vi "create initialized module for testing.vi"() -> (0 "error out":errorcluster, 1 "2d channels":refnum<class "Profibus channel.lvclass">[][](array[class]), 2 "1d channels":refnum<class "Profibus channel.lvclass">[](array[class]), 3 "Profibus Module configuration out":refnum<class "Profibus Module configuration.lvclass">, 4 "byte orders":T1[](array[typedef])=[{"slave"=1, "big endian"=TRUE}, {"slave"=2, "big endian"=FALSE}, {"slave"=5, "big endian"=TRUE}], 5 "2d names":string[][](array[string]), 6 "slave diagnostics":T2[](array[typedef]), 7 "1d names":string[](array[string]), 8 "RIO interface":string="asd")   [LabVIEW 2013, in "Profibus Module tests.lvlib"]
uses:
  Profibus Module tests.lvlib
  channel/Profibus channel.lvclass
  configuration/Profibus Module configuration.lvclass
  configuration/slave diagnostic configuration.ctl
  <vilib>/NI/Tag Bus Module Framework/channel/TBM channel.lvclass
  configuration/error throw specification.ctl
  configuration/endianness setting.ctl
  <vilib>/NI/Tag Bus/tag/Data Type.ctl
  <vilib>/NI/Tag Bus Module Framework/channel/channel classification.ctl
  configuration/Profibus Module configuration.lvclass/Profibus Module configuration.ctl
  configuration/Write RIO interface.vi
  configuration/Write slave diagnostics.vi
  configuration/Write byte orders.vi
  <vilib>/NI/Tag Bus/tag/tag descriptor.lvclass
  <vilib>/NI/Configuration Framework/serializable configuration/NISE_CEF_serializable configuration.lvclass
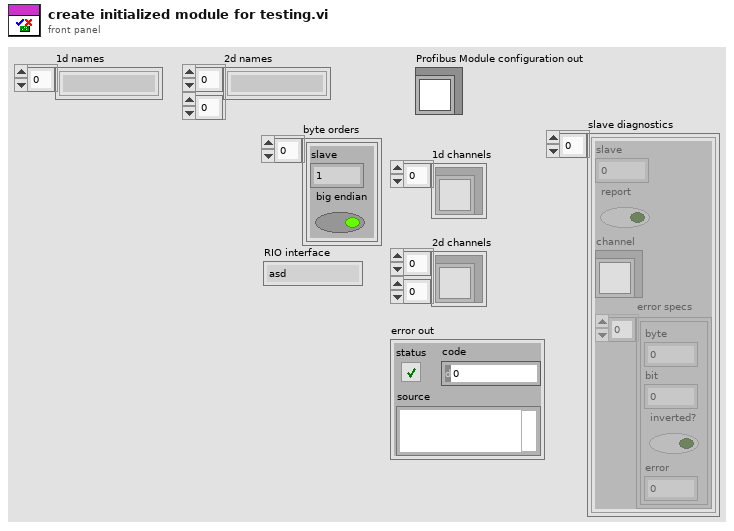
[diagram p1: front panel]
types:
  T1 = typedef "Profibus Module configuration.lvclass/endianness setting.ctl" = cluster{"slave":i8, "big endian":bool}
  T2 = typedef "Profibus Module configuration.lvclass/slave diagnostic configuration.ctl" = cluster{"slave":i8, "report":bool, "channel":refnum<class "TBM channel.lvclass">, "error specs":T3[]}
  T3 = typedef "Profibus Module configuration.lvclass/error throw specification.ctl" = cluster{"byte":i32, "bit":i32, "inverted?":bool, "error":i32}
  T4 = typedef "TBM channel.lvclass/channel classification.ctl" = enum16{"input data", "output data", "processing parameter", "processing result"}
  T5 = typedef "tag bus.lvlib/tag descriptor.lvclass/Data Type.ctl" = enum16{"Double", "Single", "I64", "I32", "I16", "I8", "U64", "U32", "U16", "U8", "Boolean", "String", "Array of Double", "Array of Single", "Array of I64", "Array of I32", "Array of I16", "Array of I8", "Array of U64", "Array of U32", "Array of U16", "Array of U8", "Array of Boolean", "Array of String"}
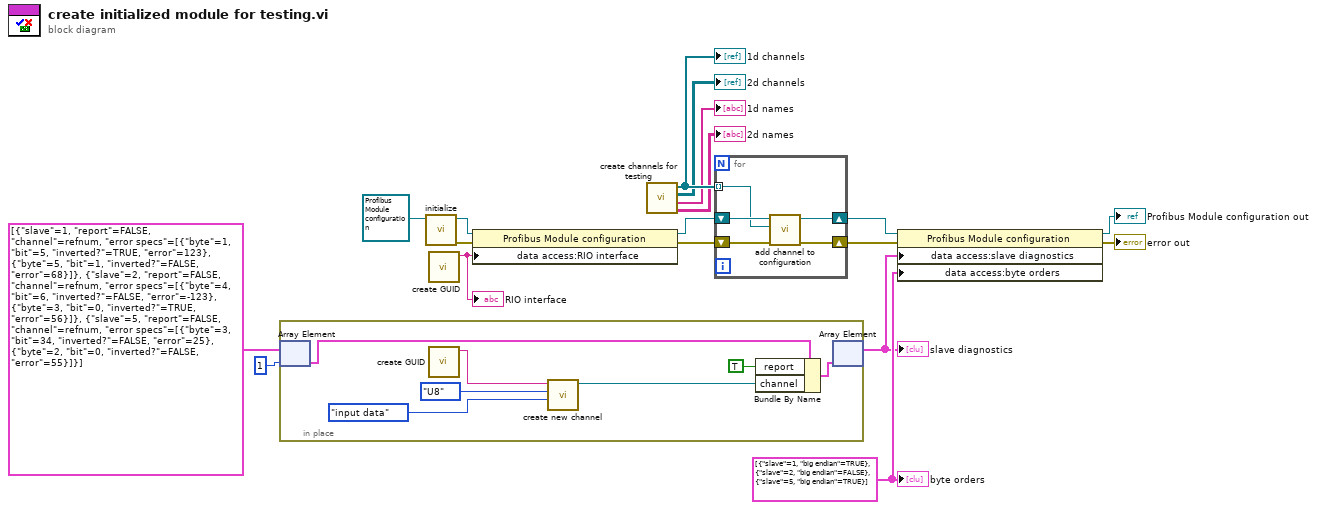
[diagram p0: block diagram]
diagram:
  w5 = T1[] [{"slave"=1, "big endian"=TRUE}, {"slave"=2, "big endian"=FALSE}, {"slave"=5, "big endian"=TRUE}] ("byte orders")
  n1 = in-place {
    n2 = in-place-array #1(T2[] [{"slave"=1, "report"=FALSE, "channel"=refnum, "error specs"=[{"byte"=1, "bit"=5, "inverted?"=TRUE, "error"=123}, {"byte"=5, "bit"=1, "inverted?"=FALSE, "error"=68}]}, {"slave"=2, "report"=FALSE, "channel"=refnum, "error specs"=[{"byte"=4, "bit"=6, "inverted?"=FALSE, "error"=-123}, {"byte"=3, "bit"=0, "inverted?"=TRUE, "error"=56}]}, {"slave"=5, "report"=FALSE, "channel"=refnum, "error specs"=[{"byte"=3, "bit"=34, "inverted?"=FALSE, "error"=25}, {"byte"=2, "bit"=0, "inverted?"=FALSE, "error"=55}]}] ("slave diagnostics"), 1) -> (w25:T2)
    n3 = call <vilib>:"create GUID.vi"() -> ("uuid"=w21:string)  [unwired: 10 in, 1 out]
    n4 = call <vilib>:"create new channel.vi"("channel classification"=channel_classification."input data", "data type"=Data_Type."U8", "channel name"=w21) -> ("channel"=w23:refnum<class "TBM channel.lvclass">)  [unwired: 8 in]
    n5 = Bundle By Name(cluster=w25, "report"=TRUE, "channel"=w23) -> (w24:T2)
    n6 = in-place-array #1(w24) -> (w3:T2[])  [unwired: 1 out]
  }
  "slave diagnostics" <- w3
  n7 = call <vilib>:"initialize.vi"("configuration in"=refnum<class "Profibus Module configuration.lvclass"> refnum ("tag bus configurable plugin module configuration")) -> ("error out"=w17:errorcluster, "configuration out"=w10:refnum<class "Profibus Module configuration.lvclass">)  [unwired: 8 in, 1 out]
  n8 = call <vilib>:"create GUID.vi"() -> ("uuid"=w1:string)  [unwired: 10 in, 1 out]
  "RIO interface" <- w1
  n9 = property class="Profibus Module configuration"(reference=w10, error in=w17, "data access:RIO interface"=w1) -> (reference out=w9:refnum<class "Profibus Module configuration.lvclass">, error out=w11:errorcluster)
  n10 = call "create channels for testing.vi"() -> ("2d names"=→"2d names":string[][], "1d names"=→"1d names":string[], "2d channels"=→"2d channels":refnum<class "Profibus channel.lvclass">[][], "1d channels"=w18:refnum<class "Profibus channel.lvclass">[])  [unwired: 8 in]
  "1d channels" <- w18
  n11 = for {
    tunnel: w18 -> [w28] mode=indexing
    shift-right: [w27] -> w7
    shift-left: w9 -> [w30]
    shift-right: [w26] -> w15
    shift-left: w11 -> [w29]
    n12 = call "add channel to configuration.vi"("error in"=w29, "TBM channel in"=w28, "Profibus Module configuration in"=w30) -> ("error out"=w26:errorcluster, "Profibus Module configuration out"=w27:refnum<class "Profibus Module configuration.lvclass">)  [unwired: 7 in]
  }
  n13 = property class="Profibus Module configuration"(reference=w7, error in=w15, "data access:slave diagnostics"=w3, "data access:byte orders"=w5) -> (reference out=→"Profibus Module configuration out":refnum<class "Profibus Module configuration.lvclass">, error out=→"error out":errorcluster)
  "byte orders" <- w5
